vi "test_config.vi"(7 "LabVIEW Web Service Request":refnum<class "Web Request.lvclass">, 11 "context_id":string) -> (2 "error_messages":string[](array[string]), 3 "valid":bool)   [LabVIEW 2013]
uses:
  <vilib>/wsapi/Web Request.lvclass
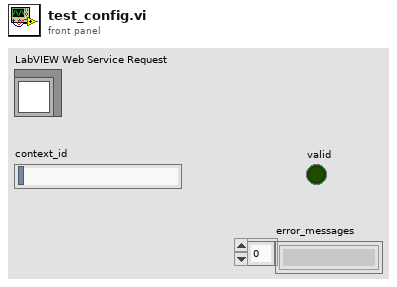
[diagram p1: front panel]
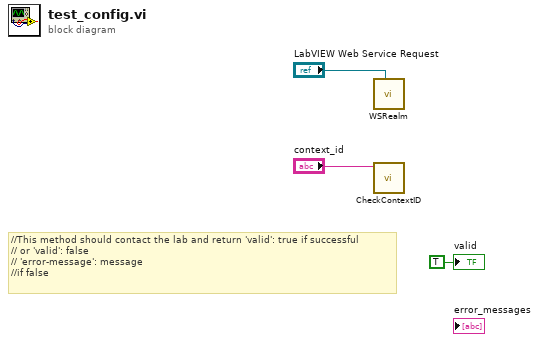
[diagram p0: block diagram]
diagram:
  # "//This method should contact the lab and return 'valid': true if successful\n// or 'valid': false\n// 'error-message': message\n//if false"
  n1 = call "WSRealm.vi"("LabVIEW Web Service Request"="LabVIEW Web Service Request") -> ()  [unwired: 11 in]
  n2 = call "CheckContextID.vi"("context_id"="context_id") -> ()  [unwired: 10 in, 1 out]
  "valid" <- TRUE ("valid")
